vi "GPIB_autodetect.vi"(8 "error in (no error)":errorcluster, 9 "Verify GPIB address":bool, 10 "Instrument GPIB address in":string, 11 "InstrControl in":refnum<class "InstrControl.lvclass">) -> (0 "error out":errorcluster, 2 "Instrument GPIB address":string, 3 "InstrControl out":refnum<class "InstrControl.lvclass">)   [LabVIEW 2019, in "InstrControl.lvclass"]
uses:
  InstrControl.lvclass
panel:
  out "instrument responses":string[](array[string])
  out "GPIB addresses found":string[](array[string])
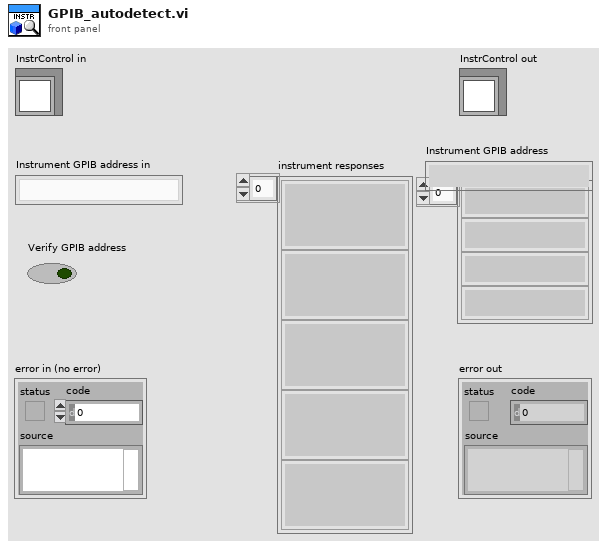
[diagram p1: front panel]
types:
  T1 = cluster{"error":bool, "code":i32, "source":string}
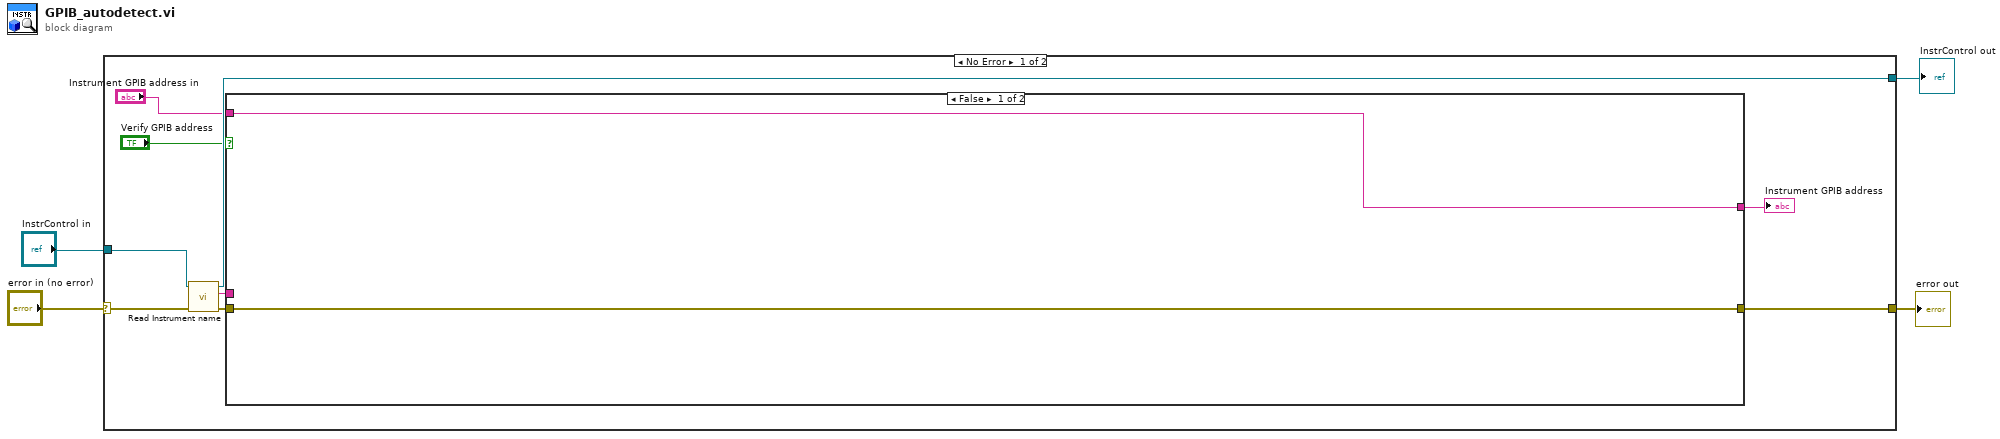
[diagram p0: block diagram]
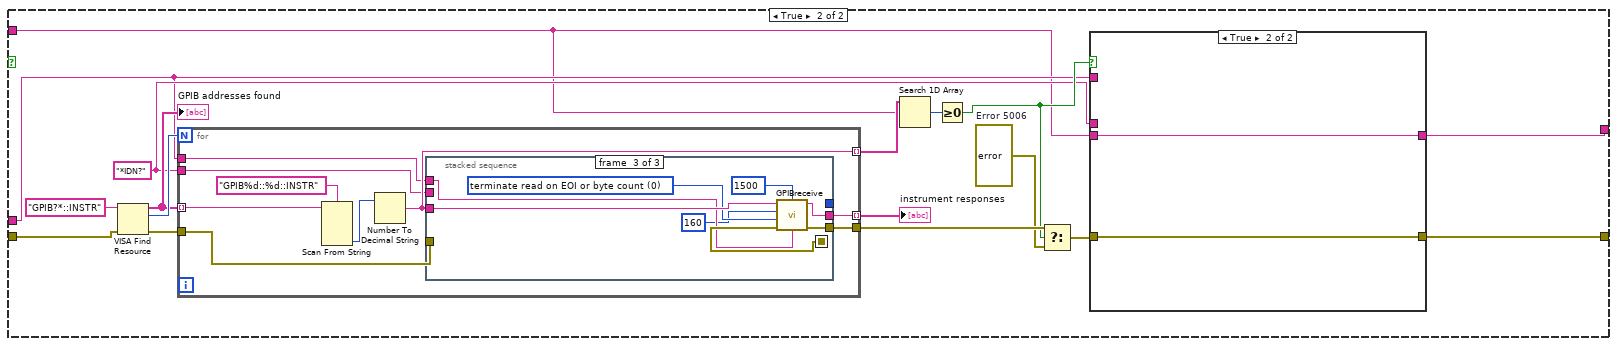
[diagram p2: hidden frame]
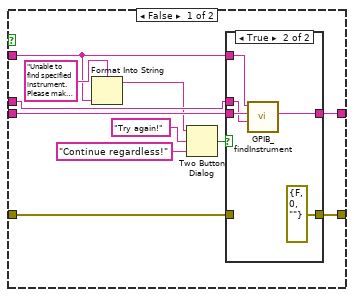
[diagram p3: hidden frame]
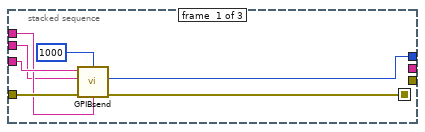
[diagram p5: hidden frame]
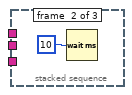
[diagram p6: hidden frame]
diagram:
  n1 = case shown="No Error" "error in (no error)" {
    selector: "error in (no error)" -> [w12 w79]
    tunnel: [w9 w79] -> w3
    tunnel: [w11 w78] -> w1
    tunnel: "InstrControl in" -> [w13 w78]
    frame No Error {
      n2 = call-dynamic "Read Instrument name.vi"("error in (no error)"=w12, "InstControl in"=w13) -> ("error out"=w10:errorcluster, "Instrument name"=w8:string, "InstControl out"=w11:refnum<class "InstrControl.lvclass">)  [unwired: 7 in]
      n3 = case shown="False" "Verify GPIB address" {
        tunnel: w10 -> [w15 w26]
        tunnel: [w15 w20] -> w9
        tunnel: w8 -> [_ w18]
        tunnel: "Instrument GPIB address in" -> [w14 w17]
        tunnel: [w14 w16] -> w5
        frame False {
        }
        frame True {
          w19 = "*IDN?" ("regular expression")
          w31 = errorcluster {"status"=FALSE, "code"=5005, "source"="Unable to find specified instrument.  Please make sure the it is connected to your system and switched on."}  # Error 5006
          n4 = VISA Find Resource(8:w26, 11:"GPIB?*::INSTR" ("expression (\"\")")) -> (0:w30:errorcluster, 2:w29:u32, 3:w28:string[])  [unwired: 1 in]
          "GPIB addresses found" <- w28
          n5 = for {
            N: w29 -> [_]
            tunnel: w28 -> [w59] mode=indexing
            tunnel: w30 -> [w61]
            tunnel: [w60] -> w32
            tunnel: [w56] -> w24 mode=indexing
            tunnel: w18 -> [w55]
            tunnel: [w57] -> w27 mode=indexing
            tunnel: w19 -> [w54]
            n6 = Scan From String(format string="GPIB%d::%d::INSTR" ("expression (\"\")"), input string=w59) -> (output 2=w53:i32)  [unwired: 5 in, 3 out]
            n7 = Number To Decimal String(number=w53) -> (decimal integer string=w56:string)  [unwired: 1 in]
            n8 = stacked-sequence {
              seq-local: [w66 _ _] -> [_ _ w76]
              tunnel: w56 -> [w68 _ w75]
              tunnel: w61 -> [w67 _ _]
              tunnel: [_ _ w77] -> w60
              tunnel: [_ _ w72] -> w57
              tunnel: w55 -> [w64 _ w73]
              tunnel: w54 -> [w63 _ _]
              tunnel: [w62 _ _] -> _
              frame #0 {
                n9 = call "GPIBsend.vi"("timeout ms"=u32 1000, "address string"=w68, "write buffer"=w63, "source"=w64, "error in"=w67) -> ("byte count"=w62:i32, "error out"=w66:errorcluster)  [unwired: 2 in, 1 out]
              }
              frame #1 {
                n10 = Wait (ms)(milliseconds to wait=10) -> ()  [unwired: 1 out]
              }
              frame #2 {
                w71 = 0 items=["terminate read on EOI or byte count", "terminate read on EOI, byte count, or CR", "terminate read on EOI, byte count, or LF"] ("read mode")
                n11 = call "GPIBreceive.vi"("timeout ms"=u32 1500, "address string"=w75, "byte count"=160, "source"=w73, "read mode"=w71, "error in"=w76) -> ("read buffer"=w72:string, "error out"=w77:T1)  [unwired: 1 in, 1 out]
              }
            }
          }
          "instrument responses" <- w27
          n12 = Search 1D Array(1D array=w24, element=w17) -> (index of element=w23:i32)  [unwired: 1 in]
          n13 = Greater Or Equal To 0?(x=w23) -> (x >= 0?=w22:bool)
          n14 = Select(t=w32, s=w22, f=w31) -> (s? t:f=w21:errorcluster)
          n15 = case shown="True" w22 {
            tunnel: w17 -> [w40 w52]
            tunnel: [w39 w52] -> w16
            tunnel: w21 -> [w38 w51]
            tunnel: [w37 w51] -> w20
            tunnel: w19 -> [w36 _]
            tunnel: w18 -> [w34 _]
            frame False {
              n16 = Format Into String(format string="Unable to find specified instrument.  Please make sure the it is connected to your system and switched on.\n\n%s" ("source"), w34) -> (resulting string=w33:string)  [unwired: 2 in, 1 out]
              n17 = Two Button Dialog(message=w33, 1:"Continue regardless!", 2:"Try again!") -> (T button?=w41:bool)
              n18 = case shown="True" w41 {
                tunnel: w40 -> [w45 w50]
                tunnel: [w45 w49] -> w39
                tunnel: w38 -> [w44 _]
                tunnel: [w44 errorcluster {"status"=FALSE, "code"=0, "source"=""} ("error constant")] -> w37
                tunnel: w36 -> [_ w47]
                tunnel: w34 -> [_ w46]
                frame False {
                }
                frame True {
                  n19 = call "GPIB_findInstrument.vi"("ID command"=w47, "revised GPIB address"=w50, "Instrument name IN"=w46) -> ("revised GPIB address OUT"=w49:string)  [unwired: 8 in]
                }
              }
            }
            frame True {
            }
          }
        }
      }
      "Instrument GPIB address" <- w5
    }
    frame Error {
    }
  }
  "error out" <- w3
  "InstrControl out" <- w1
